vi "test3-MacroWithSubAndPostMessages.vi"(8 "error in":errorcluster, 11 "TestCase in":refnum<class "testcase-CSMResponse.lvclass">) -> (0 "error out":errorcluster, 3 "TestCase out":refnum<class "testcase-CSMResponse.lvclass">)   [LabVIEW 2017, in "testcase-CSMResponse.lvclass"]
uses:
  testcase-CSMResponse.lvclass
  0c6454a9-3719-4e31-9ff6-45b39d38beb6.vi
  2437fcdf-222d-44ea-9250-34e015767128.vi
  src/user.lib/_NEVSTOP/Communicable State Machine(CSM)/AdvanceAPI/CSM - Get Module Attribute.vi
  <vilib>/addons/_JKI Toolkits/VI Tester/TestCase.llb/TestCase.lvclass
  src/user.lib/_NEVSTOP/Communicable State Machine(CSM)/Communicable State Machine.lvlib
  C:/Program Files (x86)/National Instruments/LabVIEW 2017/vi.lib/addons/_JKI Toolkits/VI Tester/TestCase.llb/TestCase.lvclass
panel:
  out "Loopcount":i32
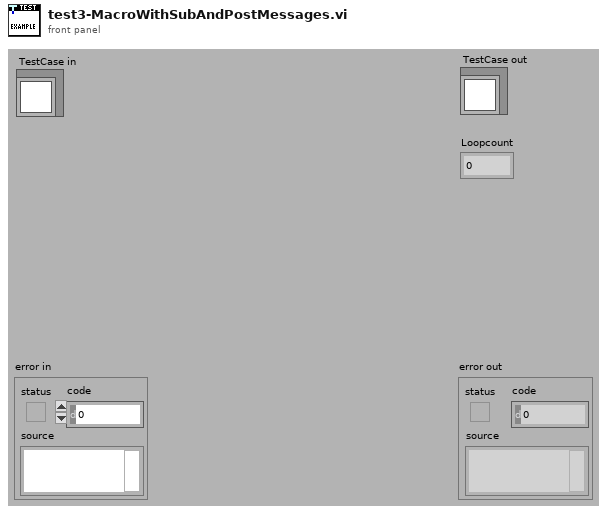
[diagram p1: front panel]
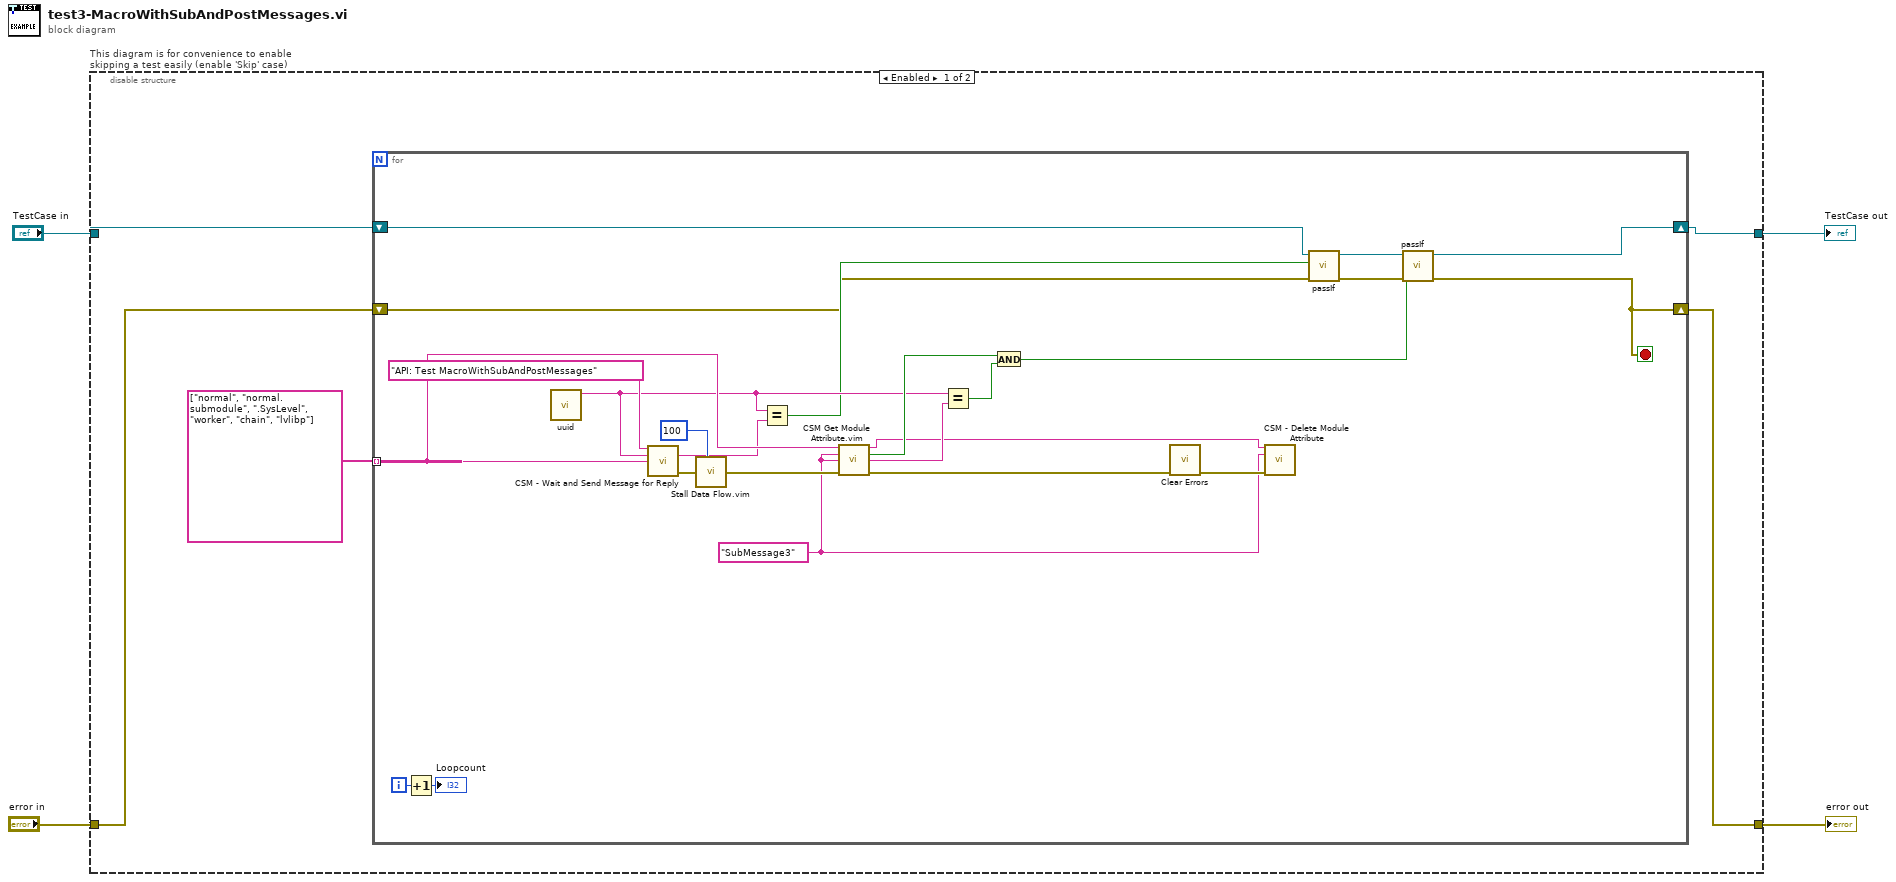
[diagram p0: block diagram]
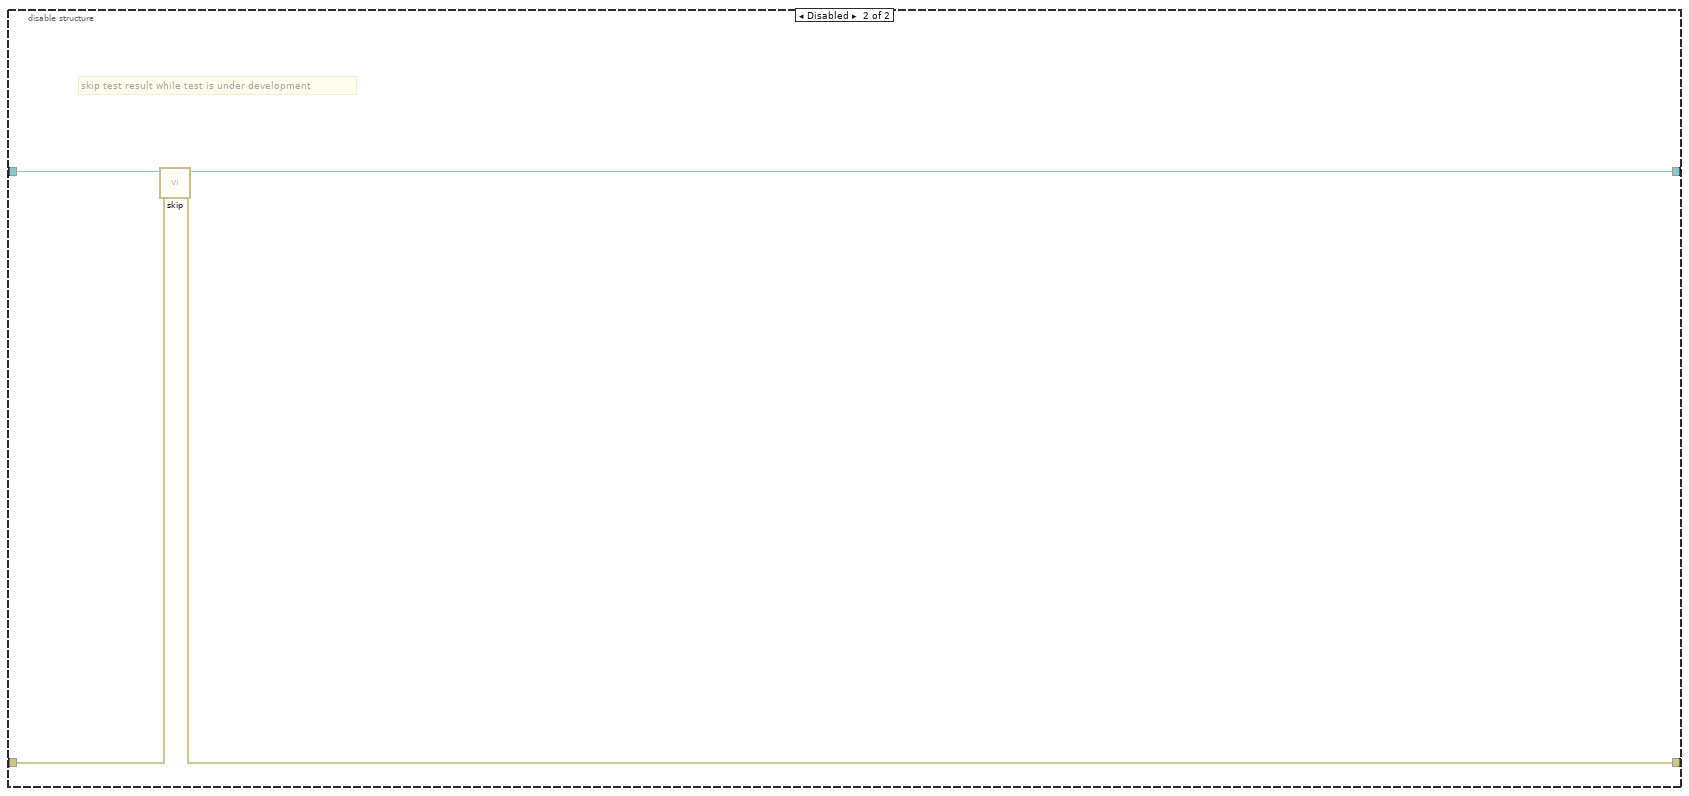
[diagram p2: hidden frame]
diagram:
  n1 = disable-structure "This diagram is for convenience to enable skipping a test easily (enable 'Skip' case)" shown="Enabled" {
    disable-tunnel: "TestCase in" -> [w9 w37]
    disable-tunnel: [w8 w35] -> w1
    disable-tunnel: [w7 w36] -> w3
    disable-tunnel: "error in" -> [w6 w34]
    frame Enabled {
      n2 = for {
        tunnel: string[] ["normal", "normal.submodule", ".SysLevel", "worker", "chain", "lvlibp"] -> [w28] mode=indexing
        shift-right: [w18] -> w8
        shift-left: w9 -> [w12]
        shift-right: [w17] -> w7
        shift-left: w6 -> [w11]
        i -> [w33]
        stop <- w17 stop-if-true
        w19 = "SubMessage3" ("Attribute")
        n3 = Increment(x=w33) -> (x+1=→"Loopcount":i32)
        n4 = call "uuid.vi"() -> ("UUID"=w15:string)  [unwired: 11 in]
        n5 = call "CSM - Wait and Send Message for Reply.vi"("State"="API: Test MacroWithSubAndPostMessages", "Arguments (\"\")"=w15, "Target Module"=w28) -> ("Response"=w16:string, "error out"=w31:errorcluster)  [unwired: 10 in, 1 out]
        n6 = call "Stall Data Flow.vim"("value in"=w31, "milliseconds to wait"=u32 100) -> ("value out"=w29:errorcluster)  [unwired: 1 out]
        n7 = Equal?(x=w15, y=w16) -> (x = y?=w14:bool)
        n8 = call "CSM Get Module Attribute.vim"("CSM Name"=w28, "Attribute"=w19, "Default Value (Empty Variant)"=w19, "Error In"=w29) -> ("CSM Name (Dup)"=w20:string, "Found"=w27:bool, "Value"=w26:string, "error out"=w22:errorcluster)  [unwired: 7 in, 1 out]
        n9 = Equal?(x=w15, y=w26) -> (x = y?=w24:bool)
        n10 = And(x=w27, y=w24) -> (x .and. y?=w23:bool)
        n11 = call <vilib>:"Clear Errors.vi"("error in (no error)"=w22) -> ("error out"=w21:errorcluster)  [unwired: 5 in, 1 out]
        n12 = call "CSM - Delete Module Attribute.vi"("CSM Name"=w20, "Attribute"=w19, "Error In"=w21) -> ()  [unwired: 9 in, 4 out]
        n13 = call-dynamic "passIf.vi"("error in (no error)"=w11, "pass"=w14, "TestCase in"=w12) -> ("error out"=w10:errorcluster, "TestCase out"=w13:refnum<class "testcase-CSMResponse.lvclass">)  [unwired: 7 in]
        n14 = call-dynamic "passIf.vi"("error in (no error)"=w10, "pass"=w23, "TestCase in"=w13) -> ("error out"=w17:errorcluster, "TestCase out"=w18:refnum<class "testcase-CSMResponse.lvclass">)  [unwired: 7 in]
      }
    }
    frame Disabled {
      # "skip test result while test is under development"
      n15 = call <vilib>:"skip.vi"("error in (no error)"=w34, "TestCase in"=w37) -> ("error out"=w36:errorcluster, "TestCase out"=w35:refnum<class "testcase-CSMResponse.lvclass">)  [unwired: 8 in]
    }
  }
  "error out" <- w3
  "TestCase out" <- w1
